vi "setCost.vi"(8 "error in (no error)":errorcluster, 10 "cost":dbl, 11 "DarkRoast in":refnum<class "DarkRoast.lvclass">) -> (0 "error out":errorcluster, 3 "DarkRoast out":refnum<class "DarkRoast.lvclass">)   [LabVIEW 2018, in "DarkRoast.lvclass"]
uses:
  DarkRoast.lvclass
  Beverage Class/Beverage.lvclass
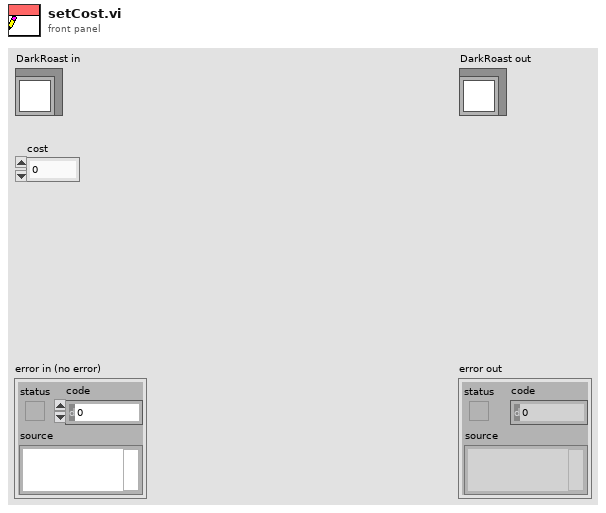
[diagram p1: front panel]
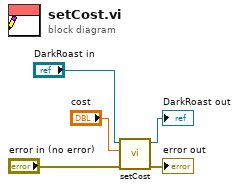
[diagram p0: block diagram]
diagram:
  n1 = call-parent "setCost.vi"("error in (no error)"="error in (no error)", "cost"="cost", "Beverage in"="DarkRoast in") -> ("error out"=→"error out":errorcluster, "Beverage out"=→"DarkRoast out":refnum<class "DarkRoast.lvclass">)  [unwired: 7 in]
